vi "Configure SPI Trigger Signals.vi"(0 "VISA resource name":refnum<visa-resource-name>, 5 "Clock Source (0: Channel 1)":u16(ring) items=["Channel 1", "Channel 2", "Channel 3", "Channel 4", "DIG 0", "DIG 1", "DIG 2", "DIG 3", "DIG 4", "DIG 5", "DIG 6", "DIG 7", "DIG 8", "DIG 9", "DIG 10", "DIG 11", "DIG 12", "DIG 13", "DIG 14", "DIG 15", "External"], 7 "Data Source (1: Channel 2)":u16(ring)=1 items=["Channel 1", "Channel 2", "Channel 3", "Channel 4", "DIG 0", "DIG 1", "DIG 2", "DIG 3", "DIG 4", "DIG 5", "DIG 6", "DIG 7", "DIG 8", "DIG 9", "DIG 10", "DIG 11", "DIG 12", "DIG 13", "DIG 14", "DIG 15", "External"], 9 "Slope (1: Positive)":u16(ring)=1 items=["Negative", "Positive"], 11 "error in (no error)":errorcluster, 12 "Frame by (0: Not Chip Select)":u16(ring) items=["Not Chip Select", "Chip Select", "Clock Timeout"], 13 "Frame Source (2: Channel 3)":u16(ring)=2 items=["Channel 1", "Channel 2", "Channel 3", "Channel 4", "DIG 0", "DIG 1", "DIG 2", "DIG 3", "DIG 4", "DIG 5", "DIG 6", "DIG 7", "DIG 8", "DIG 9", "DIG 10", "DIG 11", "DIG 12", "DIG 13", "DIG 14", "DIG 15", "External"], 14 "Timeout (10E-6)":dbl=1e-05 format="%^#_6g") -> (4 "VISA resource name out":refnum<visa-resource-name>, 15 "error out":errorcluster)   [LabVIEW 2017, in "Agilent 6000 Series.lvlib"]
doc: "This VI configures the SPI trigger. You specify the clock source, slope, data source, frame by and frame source with the Clock Source, Slope, Data Source, Frame by and Frame Source parameters.\n\n<B>NOTE:</B>\n\nThis VI is only valid for 6000 Series models. An error will be thrown if this VI is run with 5000 Series scopes."
uses:
  <instrlib>/Agilent 6000 Series/Agilent 6000 Series.lvlib
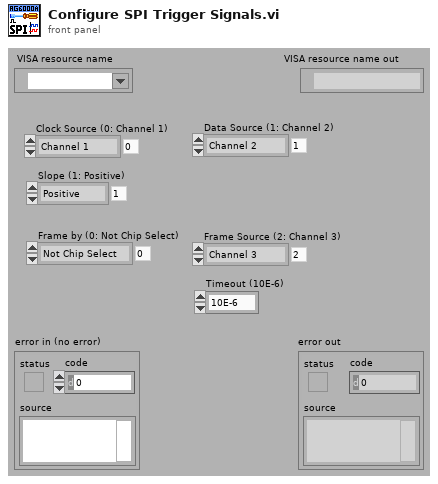
[diagram p1: front panel]
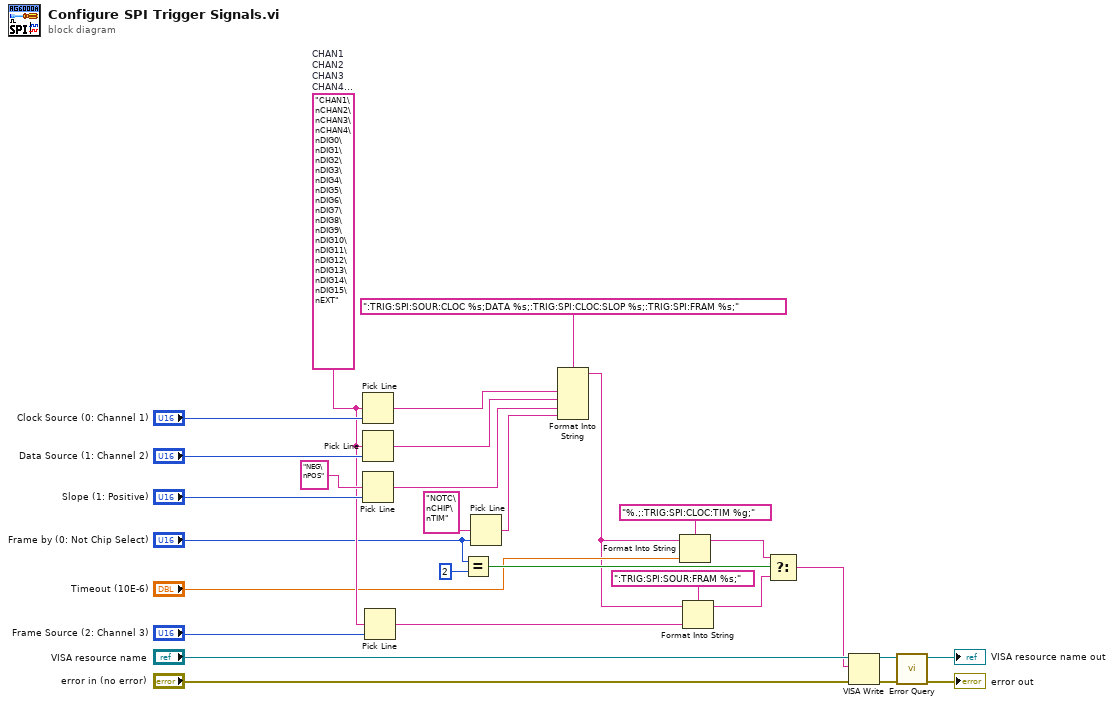
[diagram p0: block diagram]
diagram:
  w9 = "CHAN1\nCHAN2\nCHAN3\nCHAN4\nDIG0\nDIG1\nDIG2\nDIG3\nDIG4\nDIG5\nDIG6\nDIG7\nDIG8\nDIG9\nDIG10\nDIG11\nDIG12\nDIG13\nDIG14\nDIG15\nEXT"  # CHAN1 CHAN2 CHAN3 CHAN4 DIG0 DIG1 DIG2 DIG3 DIG4 DIG5 DIG6 DIG7 DIG8 DIG9 DIG10 DIG11 DIG12 DIG13 DIG14 DIG15 EXT
  n1 = Pick Line(multi-line string=w9, line index="Clock Source (0: Channel 1)") -> (output string=w16:string)  [unwired: 1 in]
  n2 = Pick Line(multi-line string=w9, line index="Data Source (1: Channel 2)") -> (output string=w14:string)  [unwired: 1 in]
  n3 = Pick Line(multi-line string="NEG\nPOS", line index="Slope (1: Positive)") -> (output string=w12:string)  [unwired: 1 in]
  n4 = Pick Line(multi-line string=w9, line index="Frame Source (2: Channel 3)") -> (output string=w7:string)  [unwired: 1 in]
  n5 = Equal?(x="Frame by (0: Not Chip Select)", y=u16 2) -> (x = y?=w19:bool)
  n6 = Pick Line(multi-line string="NOTC\nCHIP\nTIM", line index="Frame by (0: Not Chip Select)") -> (output string=w10:string)  [unwired: 1 in]
  n7 = Format Into String(format string=":TRIG:SPI:SOUR:CLOC %s;DATA %s;:TRIG:SPI:CLOC:SLOP %s;:TRIG:SPI:FRAM %s;" ("Source Command"), w16, w14, w12, w10) -> (resulting string=w2:string)  [unwired: 2 in, 1 out]
  n8 = Format Into String(format string="%.;:TRIG:SPI:CLOC:TIM %g;", initial string=w2, "Timeout (10E-6)") -> (resulting string=w5:string)  [unwired: 1 in, 1 out]
  n9 = Format Into String(format string=":TRIG:SPI:SOUR:FRAM %s;", initial string=w2, w7) -> (resulting string=w17:string)  [unwired: 1 in, 1 out]
  n10 = Select(t=w5, s=w19, f=w17) -> (s? t:f=w1:string)
  n11 = VISA Write(VISA resource name="VISA resource name", write buffer=w1, error in (no error)="error in (no error)") -> (VISA resource name out=w25:refnum<visa-resource-name>, error out=w24:errorcluster)  [unwired: 1 out]
  n12 = call <instrlib>:"Error Query.vi"("error in (no error)"=w24, "VISA resource name"=w25) -> ("error out"=→"error out":errorcluster, "VISA resource name out"=→"VISA resource name out":refnum<visa-resource-name>)  [unwired: 6 in, 2 out]
